vi "CRYShow OnOff GraphTitle.vi"(11 "DataView Array Idx":i32) -> ()   [LabVIEW 2013]
uses:
  CRYNew View Global.vi
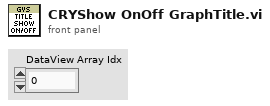
[diagram p1: front panel]
types:
  T1 = typedef "Graph Main Info Cluster.ctl" = cluster{"Selected_BarIdx":i32, "Selected_PanelIdx":i32, "Graph Main VIRef":refnum<vi>, "ToolBarClick":bool, "Spliter Ref Array":refnum<vi>[], "Panel Ref Array":refnum<vi>[], "Spliter_matrix":i32[][], "Panel_matrix":i32[][], "child_spliterIdx_matrix":i32[][], "split_pos_matrix":i32[][], "Title State":bool, "sQueueName":string, "Frame nID":i32, "Graph VIRef Array":cluster{"Graph VIRef":refnum<vi>, "Panel Idx":i32, "Frame VIRef":refnum<vi>, "Icon Ring":i32, "Graph Type":string}[], "View Type":string}
  T2 = cluster{"Graph VIRef":refnum<vi>, "Panel Idx":i32, "Frame VIRef":refnum<vi>, "Icon Ring":i32, "Graph Type":string}[]
  T3 = cluster{"Graph VIRef":refnum<vi>, "Panel Idx":i32, "Frame VIRef":refnum<vi>, "Icon Ring":i32, "Graph Type":string}
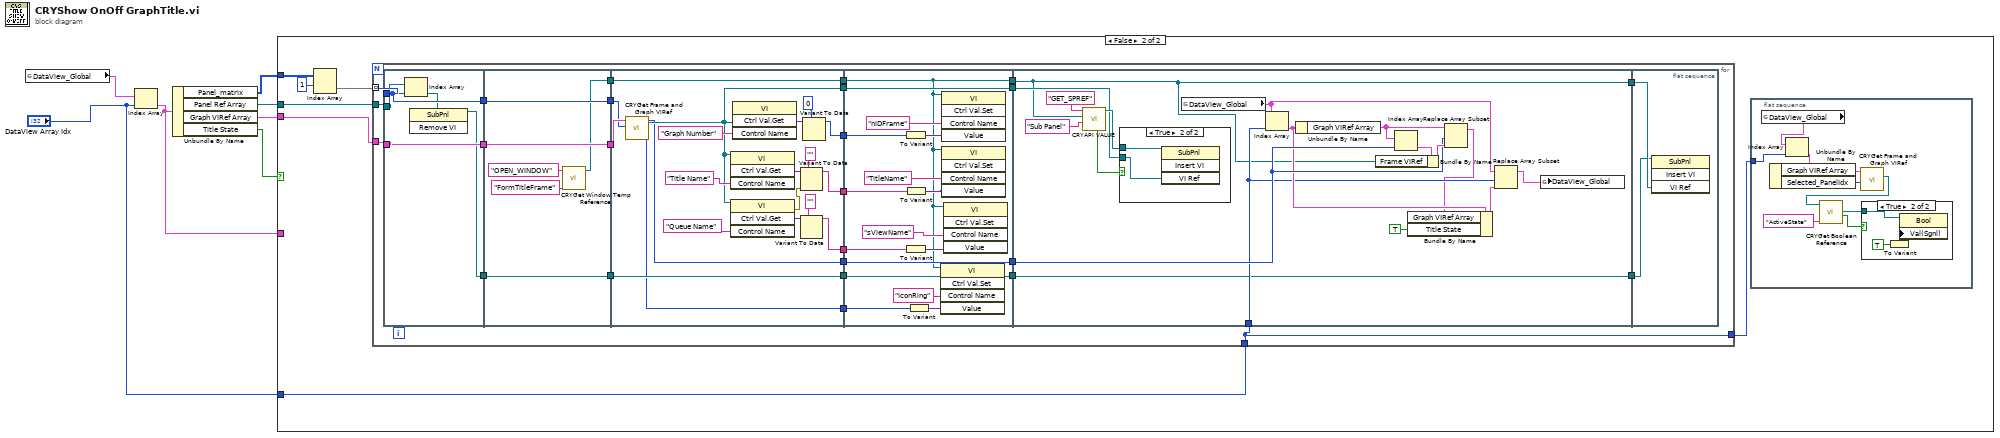
[diagram p0: block diagram]
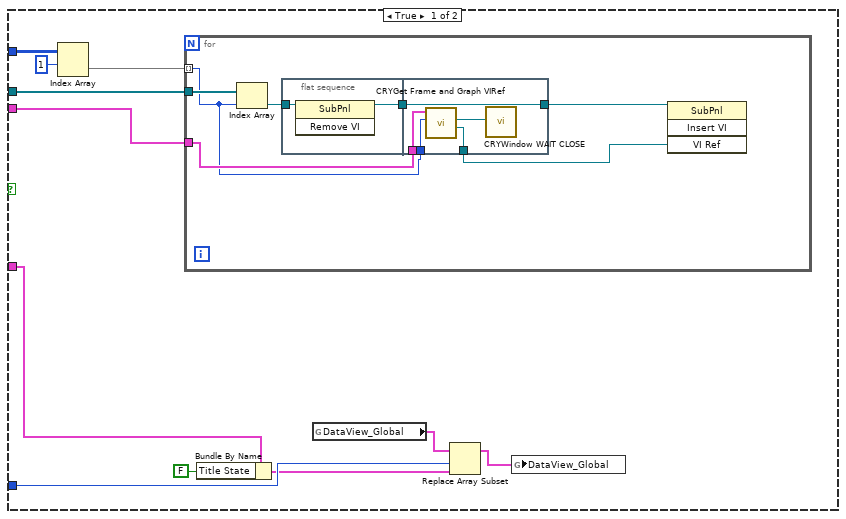
[diagram p2: hidden frame]
diagram:
  n1 = global read "CRYNew View Global.vi" "DataView_Global"() -> (w7:T1[])
  n2 = Index Array(array=w7, index="DataView Array Idx") -> (element=w1:T1)
  n3 = Unbundle By Name(w1) -> ("Panel_matrix"=w6:i32[][], "Panel Ref Array"=w5:refnum<vi>[], "Graph VIRef Array"=w4:T2, "Title State"=w3:bool)
  n4 = case shown="False" w3 {
    tunnel: w6 -> [w18 w39]
    tunnel: w5 -> [w15 w36]
    tunnel: w4 -> [w14 w35]
    tunnel: w1 -> [w13 _]
    tunnel: "DataView Array Idx" -> [w10 w34]
    frame True {
      n5 = Index Array(array=w18, index (row)=1) -> (element=w16:i32[])  [unwired: 1 in]
      n6 = for {
        tunnel: w16 -> [w20] mode=indexing
        tunnel: w15 -> [w25]
        tunnel: w14 -> [w21]
        n7 = Index Array(array=w25, index=w20) -> (element=w24:refnum<vi>)
        n8 = flat-sequence {
          tunnel: w24 -> [w27]
          tunnel: [w26] -> w22
          tunnel: [w32] -> w23
          tunnel: w22 -> [w32]
          tunnel: w21 -> [w30]
          tunnel: w20 -> [w29]
          tunnel: [w28] -> w19
          frame #0 {
            n9 = invoke class="SubPnl" method="Remove VI"(reference=w27) -> (reference out=w26:refnum<vi>)  [unwired: 2 in, 2 out]
          }
          frame #1 {
            n10 = call "CRYGet Frame and Graph VIRef.vi"("Panel Idx"=w29, "Graph VIRef Array"=w30) -> ("Graph VIRef"=w28:refnum<vi>, "Frame VIRef"=w31:refnum<vi>)  [unwired: 5 in, 3 out]
            n11 = call "CRYWindow WAIT CLOSE.vi"("vi reference"=w31) -> ()  [unwired: 11 in]
          }
        }
        n12 = invoke class="SubPnl" method="Insert VI"(reference=w23, "VI Ref"=w19) -> ()  [unwired: 2 in, 4 out]
      }
      n13 = Bundle By Name(cluster=w13, "Title State"=FALSE) -> (w9:T1)
      n14 = global read "CRYNew View Global.vi" "DataView_Global"() -> (w11:T1[])
      n15 = Replace Array Subset(array=w11, new element=w9, index=w10) -> (w8:T1[])
      n16 = global write "CRYNew View Global.vi" "DataView_Global"(w8) -> ()
    }
    frame False {
      n17 = Index Array(array=w39, index (row)=1) -> (element=w37:i32[])  [unwired: 1 in]
      n18 = for {
        tunnel: w37 -> [w75] mode=indexing
        tunnel: w36 -> [w76]
        tunnel: w35 -> [w74]
        tunnel: w34 -> [w53]
        tunnel: [w53] -> w33
        n19 = flat-sequence {
          tunnel: w76 -> [w81]
          tunnel: w75 -> [w79]
          tunnel: w74 -> [w80]
          tunnel: [w80] -> w73
          tunnel: [w79] -> w71
          tunnel: [w77] -> w58
          tunnel: w73 -> [w87]
          tunnel: [w87] -> w72
          tunnel: w71 -> [w86]
          tunnel: [w86] -> w70
          tunnel: [w83] -> w69
          tunnel: w58 -> [w82]
          tunnel: [w82] -> w54
          tunnel: w72 -> [w97]
          tunnel: w70 -> [w96]
          tunnel: w69 -> [w95]
          tunnel: [w95] -> w68
          tunnel: [w94] -> w66
          tunnel: [w93] -> w65
          tunnel: [w92] -> w64
          tunnel: [w91] -> w63
          tunnel: [w90] -> w61
          tunnel: [w89] -> w55
          tunnel: w54 -> [w89]
          tunnel: [w88] -> w52
          tunnel: w68 -> [w111]
          tunnel: [w111] -> w67
          tunnel: w66 -> [w117]
          tunnel: w65 -> [w116]
          tunnel: w64 -> [w115]
          tunnel: w63 -> [w114]
          tunnel: [w114] -> w62
          tunnel: w61 -> [w113]
          tunnel: [w113] -> w60
          tunnel: [w112] -> w56
          tunnel: w55 -> [w112]
          tunnel: w52 -> [w108]
          tunnel: w67 -> [w125]
          tunnel: w62 -> [w137]
          tunnel: w53 -> [w128]
          tunnel: w60 -> [w132]
          tunnel: [w125] -> w59
          tunnel: [w124] -> w57
          tunnel: w56 -> [w124]
          tunnel: w59 -> [w145]
          tunnel: w57 -> [w144]
          frame #0 {
            n20 = Index Array(array=w81, index=w79) -> (element=w78:refnum<vi>)
            n21 = invoke class="SubPnl" method="Remove VI"(reference=w78) -> (reference out=w77:refnum<vi>)  [unwired: 2 in, 2 out]
          }
          frame #1 {
            n22 = call "CRYGet Window Temp Reference.vi"("sWindowName"="FormTitleFrame", "sAction"="OPEN_WINDOW") -> ("pVIRef_Out"=w83:refnum<vi>)  [unwired: 5 in, 4 out]
          }
          frame #2 {
            n23 = call "CRYGet Frame and Graph VIRef.vi"("Panel Idx"=w96, "Graph VIRef Array"=w97) -> ("Icon Ring"=w88:i32, "Graph VIRef"=w91:refnum<vi>, "Graph VIRef Array Index"=w90:i32)  [unwired: 5 in, 2 out]
            n24 = invoke class="VI" method="Ctrl Val.Get"(reference=w91, "Control Name"="Title Name" ("Label Name")) -> ("Get Control Value Variant"=w101:variant)  [unwired: 2 in, 3 out]
            n25 = invoke class="VI" method="Ctrl Val.Get"(reference=w91, "Control Name"="Queue Name" ("Label Name")) -> (error out=w107:errorcluster, "Get Control Value Variant"=w106:variant)  [unwired: 2 in, 2 out]
            n26 = invoke class="VI" method="Ctrl Val.Get"(reference=w91, "Control Name"="Graph Number") -> ("Get Control Value Variant"=w99:variant)  [unwired: 2 in, 3 out]
            n27 = Variant To Data(error in=w107, type="", Variant=w101) -> (data=w93:string)  [unwired: 1 out]
            n28 = Variant To Data(type="", Variant=w106) -> (data=w92:string)  [unwired: 1 in, 1 out]
            n29 = Variant To Data(type=0, Variant=w99) -> (data=w94:i32)  [unwired: 1 in, 1 out]
          }
          frame #3 {
            n30 = To Variant(anything=w117) -> (Variant=w118:variant)
            n31 = To Variant(anything=w115) -> (Variant=w120:variant)
            n32 = To Variant(anything=w116) -> (Variant=w119:variant)
            n33 = To Variant(anything=w108) -> (Variant=w109:variant)
            n34 = invoke class="VI" method="Ctrl Val.Set"(reference=w111, "Control Name"="IconRing", "Value"=w109) -> ()  [unwired: 2 in, 5 out]
            n35 = invoke class="VI" method="Ctrl Val.Set"(reference=w111, "Control Name"="nIDFrame" ("Label Name"), "Value"=w118) -> ()  [unwired: 2 in, 5 out]
            n36 = invoke class="VI" method="Ctrl Val.Set"(reference=w111, "Control Name"="TitleName" ("Label Name"), "Value"=w119) -> ()  [unwired: 2 in, 5 out]
            n37 = invoke class="VI" method="Ctrl Val.Set"(reference=w111, "Control Name"="sViewName" ("Label Name"), "Value"=w120) -> ()  [unwired: 2 in, 5 out]
          }
          frame #4 {
            n38 = call "CRYAPI VALUE.vi"("sControlName"="Sub Panel", "pVIRef"=w125, "sAction"="GET_SPREF") -> ("pSPRef"=w138:refnum<vi>, "bResult"=w139:bool)  [unwired: 2 in, 5 out]
            n39 = case shown="True" w139 {
              tunnel: w138 -> [_ w143]
              tunnel: w137 -> [_ w142]
              frame False {
              }
              frame True {
                n40 = invoke class="SubPnl" method="Insert VI"(reference=w143, "VI Ref"=w142) -> ()  [unwired: 2 in, 4 out]
              }
            }
            n41 = global read "CRYNew View Global.vi" "DataView_Global"() -> (w131:T1[])
            n42 = Index Array(array=w131, index=w128) -> (element=w130:T1)
            n43 = Unbundle By Name(w130) -> ("Graph VIRef Array"=w133:T2)
            n44 = Index Array(array=w133, index=w132) -> (element=w135:T3)
            n45 = Bundle By Name(cluster=w135, "Frame VIRef"=w125) -> (w134:T3)
            n46 = Replace Array Subset(array=w133, new element=w134, index=w132) -> (w127:T2)
            n47 = Bundle By Name(cluster=w130, "Graph VIRef Array"=w127, "Title State"=TRUE) -> (w129:T1)
            n48 = Replace Array Subset(array=w131, new element=w129, index=w128) -> (w136:T1[])
            n49 = global write "CRYNew View Global.vi" "DataView_Global"(w136) -> ()
          }
          frame #5 {
            n50 = invoke class="SubPnl" method="Insert VI"(reference=w144, "VI Ref"=w145) -> ()  [unwired: 2 in, 4 out]
          }
        }
      }
      n51 = flat-sequence {
        tunnel: w33 -> [w47]
        frame #0 {
          n52 = global read "CRYNew View Global.vi" "DataView_Global"() -> (w48:T1[])
          n53 = Index Array(array=w48, index=w47) -> (element=w46:T1)
          n54 = Unbundle By Name(w46) -> ("Graph VIRef Array"=w45:T2, "Selected_PanelIdx"=w44:i32)
          n55 = call "CRYGet Frame and Graph VIRef.vi"("Panel Idx"=w44, "Graph VIRef Array"=w45) -> ("Frame VIRef"=w43:refnum<vi>)  [unwired: 5 in, 4 out]
          n56 = call "CRYGet Boolean Reference.vi"("Label Name"="ActiveState", "VI Refnum"=w43) -> ("Exist?"=w40:bool, "Boolean Ref"=w42:refnum<vi>)  [unwired: 7 in, 1 out]
          n57 = case shown="True" w40 {
            tunnel: w42 -> [_ w51]
            frame False {
            }
            frame True {
              n58 = To Variant(anything=TRUE) -> (Variant=w49:variant)
              n59 = property class="Bool"(reference=w51, "Val(Sgnl)"=w49) -> ()  [unwired: 1 in, 2 out]
            }
          }
        }
      }
    }
  }
